vi "01_CheckRemoteShutdown.vi"() -> ()   [LabVIEW 2020]
uses:
  librarian_class/librarian.lvclass
  client_class/client.lvclass
panel:
  out "client error out":errorcluster
  out "lib error out":errorcluster
  in  "stop":bool
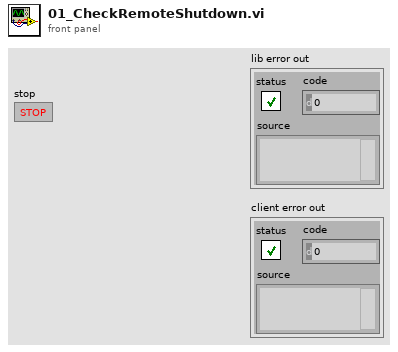
[diagram p1: front panel]
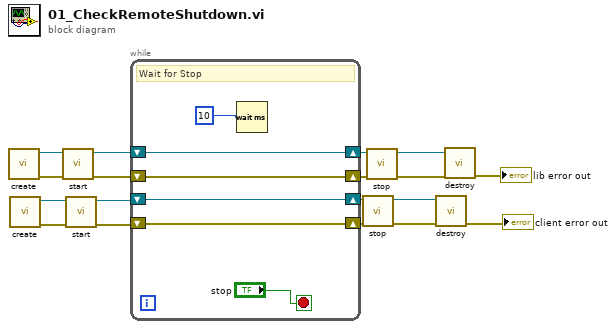
[diagram p0: block diagram]
diagram:
  n1 = call "create.vi"() -> ("error out"=w17:errorcluster, "librarian_sm out"=w18:refnum<class "librarian.lvclass">)  [unwired: 10 in]
  n2 = call "create.vi"() -> ("error out"=w8:errorcluster, "librarian_sm out"=w9:refnum<class "client.lvclass">)  [unwired: 10 in]
  n3 = call "start.vi"("error in (no error)"=w17, "librarian_sm in"=w18) -> ("error out"=w16:errorcluster, "librarian_sm out"=w15:refnum<class "librarian.lvclass">)  [unwired: 8 in]
  n4 = call "start.vi"("error in (no error)"=w8, "librarian_sm in"=w9) -> ("error out"=w6:errorcluster, "librarian_sm out"=w7:refnum<class "client.lvclass">)  [unwired: 8 in]
  n5 = while {
    shift-right: [w22] -> w14
    shift-left: w15 -> [w22]
    shift-right: [w21] -> w13
    shift-left: w16 -> [w21]
    shift-right: [w20] -> w5
    shift-left: w7 -> [w20]
    shift-right: [w19] -> w4
    shift-left: w6 -> [w19]
    stop <- "stop" stop-if-true
    # "Wait for Stop"
    n6 = Wait (ms)(milliseconds to wait=u32 10) -> ()  [unwired: 1 out]
  }
  n7 = call "stop.vi"("error in (no error)"=w4, "librarian_sm in"=w5) -> ("error out"=w2:errorcluster, "librarian_sm out"=w3:refnum<class "client.lvclass">)  [unwired: 8 in]
  n8 = call "stop.vi"("error in (no error)"=w13, "librarian_sm in"=w14) -> ("error out"=w11:errorcluster, "librarian_sm out"=w12:refnum<class "librarian.lvclass">)  [unwired: 8 in]
  n9 = call "destroy.vi"("error in (no error)"=w2, "librarian_sm in"=w3) -> ("error out"=→"client error out":errorcluster)  [unwired: 8 in, 1 out]
  n10 = call "destroy.vi"("error in (no error)"=w11, "librarian_sm in"=w12) -> ("error out"=→"lib error out":errorcluster)  [unwired: 8 in, 1 out]
